vi "MessageName.vi"() -> (2 "MessageName":string)   [LabVIEW 2020, in "TcpClientList.lvlib"]
uses:
  TcpClientList.lvlib
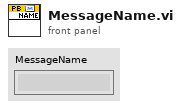
[diagram p1: front panel]
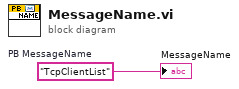
[diagram p0: block diagram]
diagram:
  w1 = "TcpClientList"  # PB MessageName
  "MessageName" <- w1
